vi "Configure Master Controller.vi"(8 "error in":errorcluster, 11 "EMS Generic in":refnum<class "EMS Generic.lvclass">) -> (0 "error out":errorcluster, 3 "EMS Generic out":refnum<class "EMS Generic.lvclass">)   [LabVIEW 2018, in "EMS Generic Actor.lvlib" / "EMS Generic.lvclass"]
doc: "This VI reads the EMS-config.ini file in the Confiuguration folder in the Application Directory and parses it for locations for device configuration files and logs."
uses:
  EMS Generic.lvclass
  EMS User Interface Actor/EMS User Interface/Controls/Configuration/File Access Command.ctl
  EMS Generic.lvclass/EMS Generic.ctl
  <vilib>/Utility/config.llb/Read Key (Path).vi
  <vilib>/Utility/config.llb/Read Key (String).vi
  <vilib>/Utility/config.llb/NI_LVConfig.lvlib
  EMS User Interface Actor/EMS User Interface/EMS User Interface.lvclass
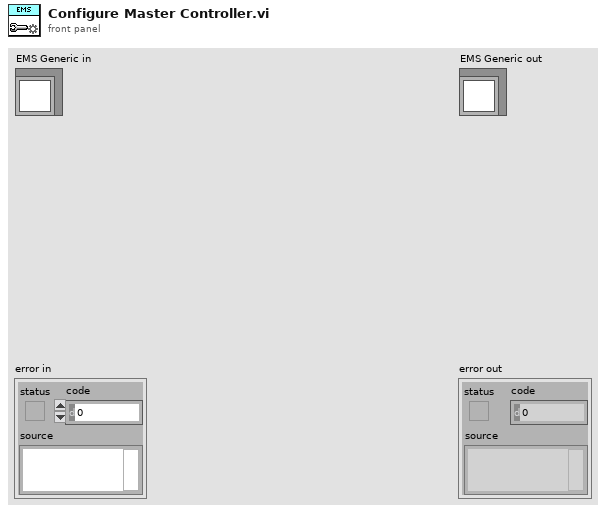
[diagram p1: front panel]
types:
  T1 = typedef "EMS User Interface Actor.lvlib/EMS User Interface.lvclass/File Access Command.ctl" = enum16{"Read", "Write"}
  T2 = typedef "NI_LVConfig.lvlib/Config Data RefNum.ctl" = refnum<k1>
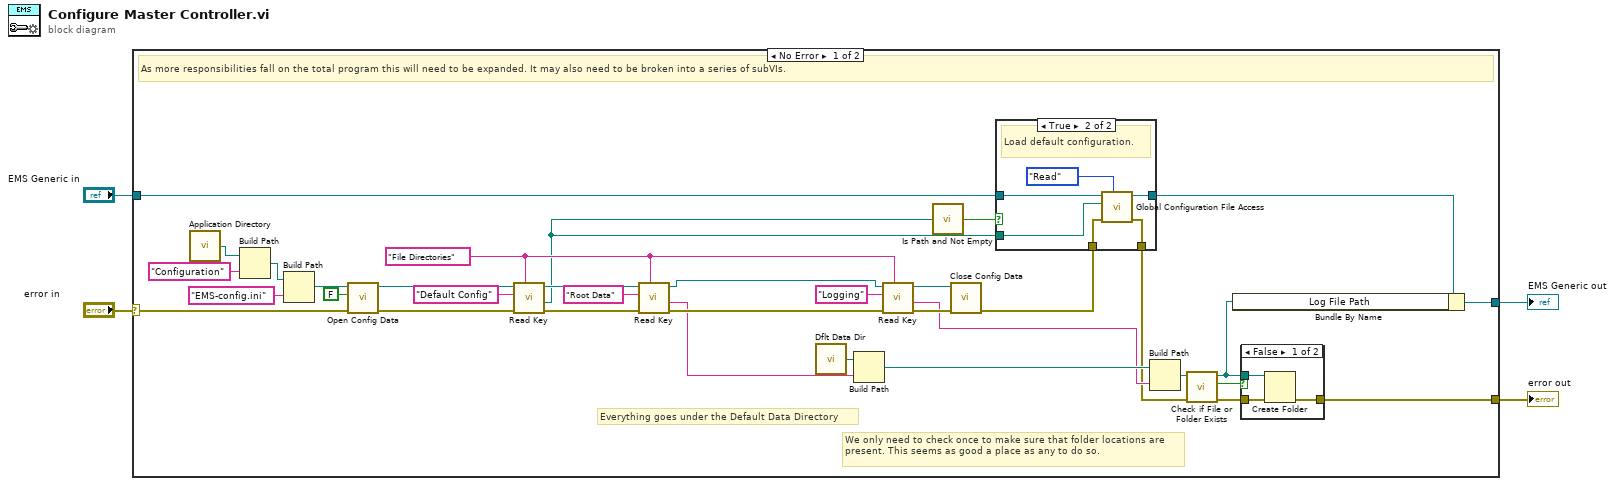
[diagram p0: block diagram]
diagram:
  n1 = case shown="No Error" "error in" {
    selector: "error in" -> [w34 w53]
    tunnel: [w19 w53] -> w3
    tunnel: [w22 w52] -> w1
    tunnel: "EMS Generic in" -> [w9 w52]
    frame No Error {
      w11 = "File Directories" ("section")
      # "Everything goes under the Default Data Directory"
      # "We only need to check once to make sure that folder locations are present. This seems as good a place as any to do so."
      # "As more responsibilities fall on the total program this will need to be expanded. It may also need to be broken into a series of subVIs."
      n2 = call <vilib>:"Application Directory.vi"() -> ("Application Directory"=w38:path)
      n3 = Build Path(base path=w38, name or relative path="Configuration") -> (appended path=w37:path)
      n4 = Build Path(base path=w37, name or relative path="EMS-config.ini") -> (appended path=w35:path)
      n5 = call <vilib>:"Open Config Data.vi"("error in (no error)"=w34, "create file if necessary (T)"=FALSE, "configuration file path"=w35) -> ("error out"=w12:errorcluster, "refnum"=w14:T2)  [unwired: 6 in, 1 out]
      n6 = call-poly <vilib>:"Read Key.vi"("section"=w11, "error in (no error)"=w12, "key"="Default Config", "refnum"=w14) -> ("error out"=w13:errorcluster, "value"=w7:path, "refnum out"=w15:T2)  [unwired: 4 in, 1 out]
      n7 = call-poly <vilib>:"Read Key.vi"("section"=w11, "error in (no error)"=w13, "key"="Root Data", "refnum"=w15) -> ("error out"=w30:errorcluster, "value"=w27:string, "refnum out"=w31:T2)  [unwired: 4 in, 1 out]
      n8 = call <vilib>:"Dflt Data Dir.vi"() -> ("App:Default Data Directory"=w28:path)
      n9 = Build Path(base path=w28, name or relative path=w27) -> (appended path=w23:path)
      n10 = call-poly <vilib>:"Read Key.vi"("section"=w11, "error in (no error)"=w30, "key"="Logging", "refnum"=w31) -> ("error out"=w18:errorcluster, "value"=w17:string, "refnum out"=w20:T2)  [unwired: 4 in, 1 out]
      n11 = call <vilib>:"Is Path and Not Empty.vi"("path"=w7) -> ("Is Path and Not Empty?"=w10:bool)  [unwired: 4 in]
      n12 = call <vilib>:"Close Config Data.vi"("error in (no error)"=w18, "refnum"=w20) -> ("error out"=w6:errorcluster)  [unwired: 8 in, 1 out]
      n13 = case shown="True" w10 {
        tunnel: w9 -> [w41 w44]
        tunnel: [w41 w47] -> w8
        tunnel: w7 -> [_ w46]
        tunnel: w6 -> [w40 w43]
        tunnel: [w40 w42] -> w5
        frame False {
          # "Do nothing"
        }
        frame True {
          # "Load default configuration."
          n14 = call "Global Configuration File Access.vi"("Command"=File_Access_Command."Read", "error in"=w43, "configuration file path"=w46, "EMS Generic in"=w44) -> ("error out"=w42:errorcluster, "EMS Generic out"=w47:refnum<class "EMS Generic.lvclass">)  [unwired: 6 in]
        }
      }
      n15 = Build Path(base path=w23, name or relative path=w17) -> (appended path=w26:path)
      n16 = call <vilib>:"Check if File or Folder Exists.vi"("error in (no error)"=w5, "path"=w26) -> ("error out"=w24:errorcluster, "file or folder exists?"=w25:bool, "dup path"=w21:path)  [unwired: 7 in]
      n17 = Bundle By Name(cluster=w8, "Log File Path"=w21) -> (w22:refnum<class "EMS Generic.lvclass">)
      n18 = case shown="False" w25 {
        tunnel: w21 -> [w50 _]
        tunnel: w24 -> [w49 w51]
        tunnel: [w48 w51] -> w19
        frame False {
          n19 = Create Folder(path (use dialog)=w50, error in=w49) -> (error out=w48:errorcluster)  [unwired: 1 in, 2 out]
        }
        frame True {
        }
      }
    }
    frame Error {
    }
  }
  "error out" <- w3
  "EMS Generic out" <- w1
